vi "Get_Available_Cameras_Direct.vi"() -> (1 "Cameras":string[](array[string]))   [LabVIEW 2020]
doc: "Self-test all hardware devices on the system specified."
uses:
  <resource>/objmgr/nisysapi.rc
  <vilib>/nisyscfg/Close (System).vi
  <vilib>/nisyscfg/Close (Filter).vi
panel:
  in  "User Name":string
  in  "Password":string
  in  "Target (localhost)":refnum<k21>="localhost"
  out "Results":string[][](table)
  # "Overview: Self-Test all hardware on the system specified.\nRequirements: NI System Configuration, applicable device drivers \nInstructions:\n1. Select Target. Enter User Name and Password if necessary.\n2. Run the VI."
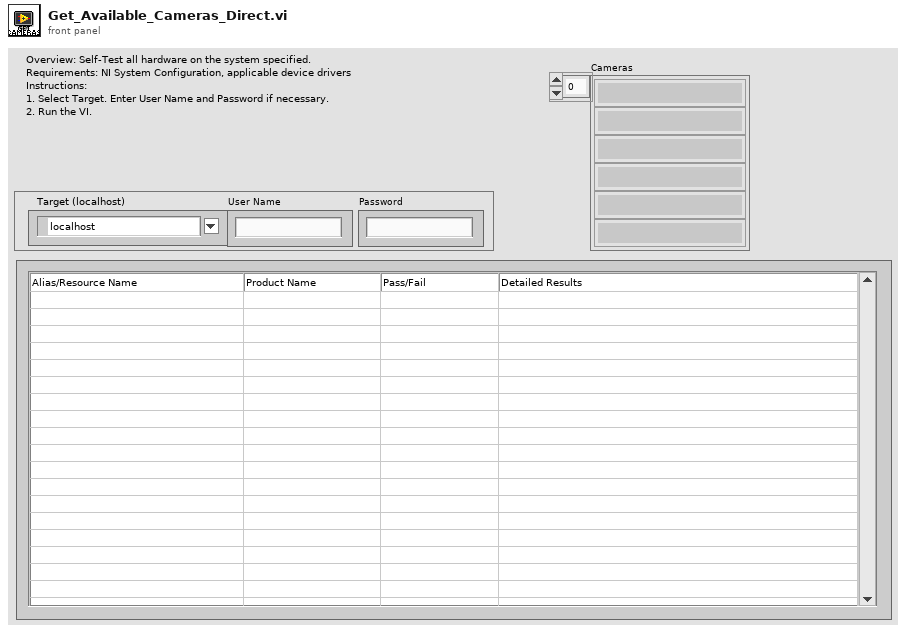
[diagram p1: front panel]
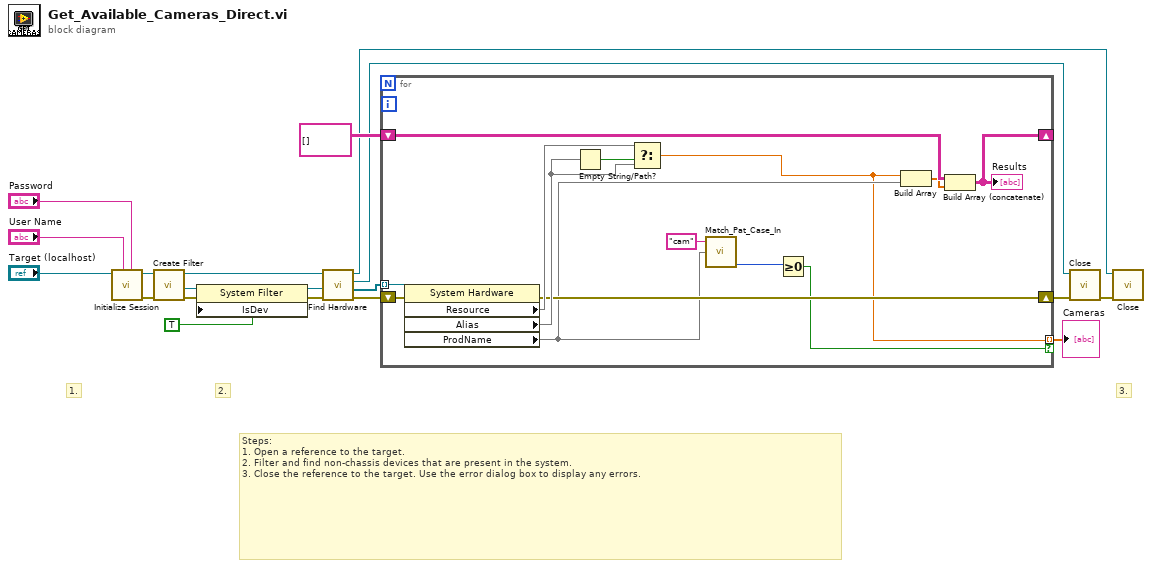
[diagram p0: block diagram]
diagram:
  # "3."
  # "2."
  # "1."
  # "Steps:\n1. Open a reference to the target.\n2. Filter and find non-chassis devices that are present in the system.\n3. Close the reference to the target. Use the error dialog box to display any errors."
  n1 = call <vilib>:"Initialize Session.vi"("Password"="Password", "User Name"="User Name", "Target (localhost)"="Target (localhost)") -> ("error out"=w15:errorcluster, "Session out"=w16:refnum<k21>)  [unwired: 7 in]
  n2 = call <vilib>:"Create Filter.vi"("error in (no error)"=w15, "Session in"=w16) -> ("error out"=w11:errorcluster, "Filter out"=w14:refnum<k20>, "Session out"=w17:refnum<k21>)  [unwired: 7 in]
  n3 = property class="System Filter"(reference=w14, error in=w11, "IsDev"=TRUE ("Is Device")) -> (reference out=w13:refnum<k20>, error out=w10:errorcluster)
  n4 = call <vilib>:"Find Hardware.vi"("error in (no error)"=w10, "Filter in"=w13, "Session in"=w17) -> ("error out"=w18:errorcluster, "Resources out"=w19:refnum<k20>[], "Filter out"=w6:refnum<k20>, "Session out"=w5:refnum<k21>)  [unwired: 1 in, 4 out]
  n5 = for {
    tunnel: w19 -> [w32] mode=indexing
    shift-right: [w29] -> _
    shift-left: string[][] [] ("appended array") -> [w30]
    shift-right: [w25] -> w7
    shift-left: w18 -> [w31]
    tunnel: [w21] -> w1 mode=indexing if=w20
    n6 = property class="System Hardware"(reference=w32, error in=w31) -> (error out=w25:errorcluster, "Resource"=w27, "Alias"=w26, "ProdName"=w23)  [unwired: 1 out]
    n7 = Empty String/Path?(string/path=w26) -> (empty?=w33:bool)
    n8 = Select(t=w27, s=w33, f=w26) -> (s? t:f=w21:dbl)
    n9 = call "Match_Pat_Case_In.vi"("String to match"="cam", "String"=w23) -> ("offset past match"=w22:i32)  [unwired: 1 in, 3 out]
    n10 = Greater Or Equal To 0?(x=w22) -> (x >= 0?=w20:bool)
    n11 = Build Array(w21, w23) -> (w28:dbl[])
    n12 = Build Array (concatenate)(w30, w28) -> (w29:string[][])
    "Results" <- w29
  }
  "Cameras" <- w1
  n13 = call-poly <vilib>:"Close.vi"("error in (no error)"=w7, "Filter in"=w6) -> ("error out"=w8:errorcluster)  [unwired: 9 in]
  n14 = call-poly <vilib>:"Close.vi"("error in (no error)"=w8, "Session in"=w5) -> ()  [unwired: 9 in, 1 out]
